vi "Version et config.vi"() -> (3 "OutPut":T1={"Date"="", "Version"="", "Titre"="", "Fichier Application"="Setting.ini"})   [LabVIEW 2020]
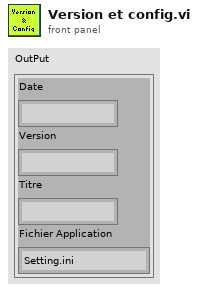
[diagram p1: front panel]
types:
  T1 = cluster{"Date":string, "Version":string, "Titre":string, "Fichier Application":string}
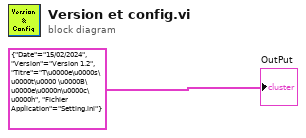
[diagram p0: block diagram]
diagram:
  "OutPut" <- T1 {"Date"="15/02/2024", "Version"="Version 1.2", "Titre"="T\u0000e\u0000s\u0000t\u0000 \u0000B\u0000e\u0000n\u0000c\u0000h", "Fichier Application"="Setting.ini"} ("OutPut")
